vi "test_calc-rotational_matrix.vi"() -> ()   [LabVIEW 2019]
uses:
  <vilib>/Analysis/coordinate.llb/Euler Rotation Order.ctl
  <vilib>/Analysis/NI_AALPro.lvlib
panel:
  out "trans2":dbl[][](array[numeric])
  out "mat":dbl[][](array[numeric]) caption="방향 코사인"
  out "trans1":dbl[][](array[numeric])
  in  "angle":dbl format="%#_13g"
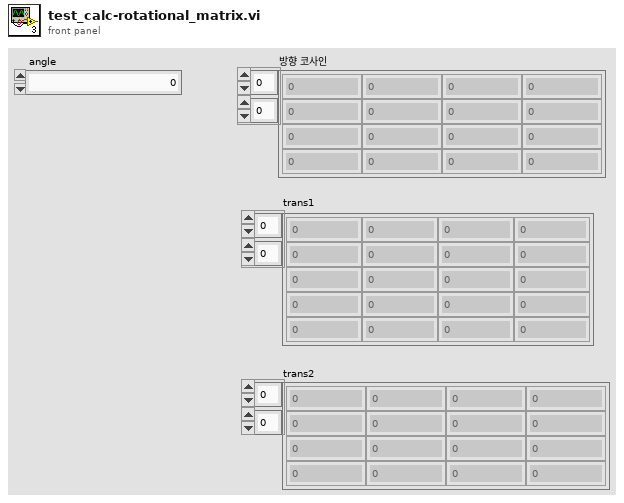
[diagram p1: front panel]
types:
  T1 = typedef "NI_AALPro.lvlib/Euler Rotation Order.ctl" = u16
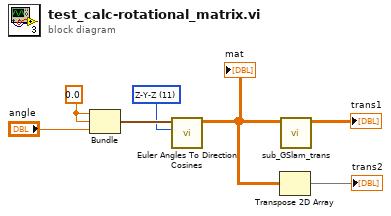
[diagram p0: block diagram]
diagram:
  w5 = T1 11 items=["X-Y-Z", "X-Z-Y", "Y-X-Z", "Y-Z-X", "Z-X-Y", "Z-Y-X", "X-Y-X", "X-Z-X", "Y-X-Y", "Y-Z-Y", "Z-X-Z", "Z-Y-Z"] ("rotation order")
  w7 = 0.0 ("원소")
  n1 = Bundle("원소"=w7, "원소"=w7, "angle"="angle") -> (w6:cluster{"원소":dbl, "원소":dbl, "angle":dbl})  [unwired: 1 in]
  n2 = call <vilib>:"Euler Angles To Direction Cosines.vi"("rotation order"=w5, "Euler Angles"=w6) -> ("Direction Cosines"=w2:dbl[][])  [unwired: 8 in, 1 out]
  "mat" <- w2
  n3 = Transpose 2D Array(2D array=w2) -> (transposed array=→"trans2":dbl[][])
  n4 = call "sub_GSlam_trans.vi"("Direction Cosines 입력"=w2) -> ("Direction Cosines 출력"=→"trans1":dbl[][])  [unwired: 10 in]
